vi "纳清_第二点校准数据写入.vi"(7 "探头":T1(ring), 8 "error in (no error)":errorcluster caption="错误输入（无错误）", 10 "数值":sgl, 11 "MB session in":refnum<class "MB_Master.lvclass">) -> (0 "error out":errorcluster caption="错误输出", 3 "MB session out":refnum<class "MB_Master.lvclass">)   [LabVIEW 2016, in "斯坦道多参数.lvlib"]
uses:
  <vilib>/Plasmionique/MB Master/MB Master.lvlib
  <vilib>/Plasmionique/MB Master/MB_Master/MB_Master.lvclass
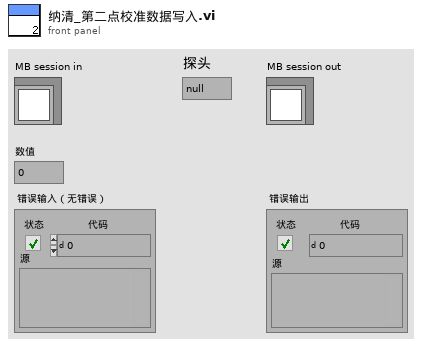
[diagram p1: front panel]
types:
  T1 = enum16{"null", "pH", "DO", "浊度", "电导率", "叶绿素a", "藻密度", "氨氮"}
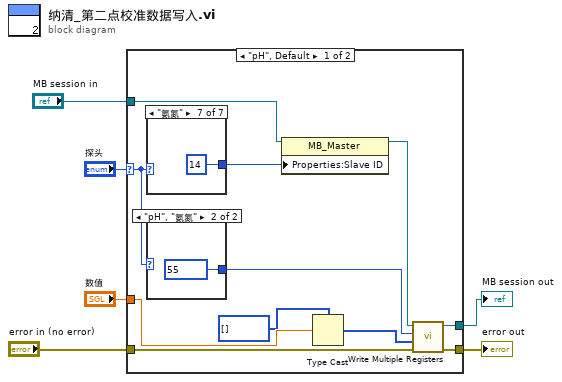
[diagram p0: block diagram]
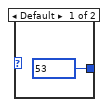
[diagram p2: hidden frame]
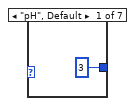
[diagram p3: hidden frame]
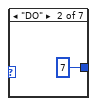
[diagram p4: hidden frame]
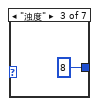
[diagram p5: hidden frame]
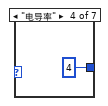
[diagram p6: hidden frame]
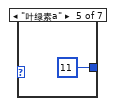
[diagram p7: hidden frame]
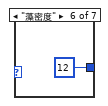
[diagram p8: hidden frame]
diagram:
  n1 = case shown="\"pH\", Default" "探头" {
    selector: "探头" -> [w7 _]
    tunnel: "error in (no error)" -> [w17 w27]
    tunnel: [w16 w27] -> w5
    tunnel: "数值" -> [w14 _]
    tunnel: "MB session in" -> [w11 w28]
    tunnel: [w10 w28] -> w2
    frame "pH", Default {
      n2 = case shown="\"氨氮\"" w7 {
        tunnel: [3 7 8 4 11 12 14] -> w9
        frame "pH", Default {
        }
        frame "DO" {
        }
        frame "浊度" {
        }
        frame "电导率" {
        }
        frame "叶绿素a" {
        }
        frame "藻密度" {
        }
        frame "氨氮" {
        }
      }
      n3 = case shown="\"pH\", \"氨氮\"" w7 {
        tunnel: [u16 53 ("starting address") u16 55 ("starting address")] -> w8
        frame Default {
        }
        frame "pH", "氨氮" {
        }
      }
      n4 = property class="MB_Master"(reference=w11, "Properties:Slave ID"=w9) -> (reference out=w15:refnum<class "MB_Master.lvclass">)  [unwired: 1 in, 1 out]
      n5 = Type Cast(type=u16[] [], x=w14) -> (*(type *) &x=w12:u16[])
      n6 = call <vilib>:"Write Multiple Registers.vi"("error in (no error)"=w17, "values"=w12, "starting address"=w8, "MB session in"=w15) -> ("error out"=w16:errorcluster, "MB session out"=w10:refnum<class "MB_Master.lvclass">)  [unwired: 6 in]
    }
    frame "null", "DO", "电导率" {
      # "电导率只有单点校准,DO无需写入校准值"
    }
  }
  "error out" <- w5
  "MB session out" <- w2
